vi "prosta najlepszego dopasowania.vi"(10 "Wartoœci Y":dbl[](array[numeric]), 11 "Wartoœci X":dbl[](array[numeric])) -> (3 "Waveform Graph":dbl[](graph))   [LabVIEW 2020]
uses:
  <vilib>/Analysis/NI_AALPro.lvlib
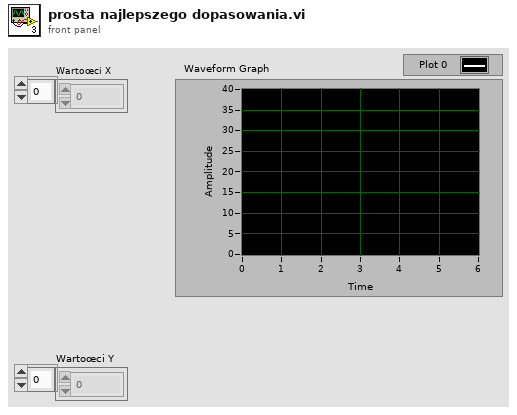
[diagram p1: front panel]
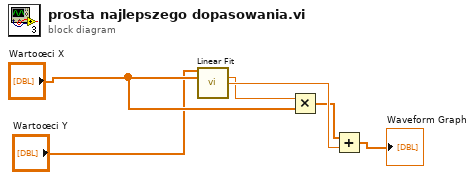
[diagram p0: block diagram]
diagram:
  n1 = call <vilib>:"Linear Fit.vi"("Y"="Wartoœci Y", "X"="Wartoœci X") -> ("slope"=w2:dbl, "intercept"=w5:dbl)  [unwired: 9 in, 3 out]
  n2 = Multiply(x=w2, y="Wartoœci X") -> (x*y=w4:dbl[])
  n3 = Add(x=w4, y=w5) -> (x+y=→"Waveform Graph":dbl[])
